vi "startup.vi"(8 "error in (no error)":errorcluster, 9 "deviceDataBase":refnum<class "deviceDataBase.lvclass">, 10 "HWControllerEvents":refnum<class "HWControllerEvents.lvclass">, 11 "Compiler in":refnum<class "Compiler.lvclass">) -> (0 "error out":errorcluster, 3 "Compiler out":refnum<class "Compiler.lvclass">)   [LabVIEW 2009, in "Compiler.lvlib" / "Compiler.lvclass"]
uses:
  Compiler.lvclass
  Hal/HWController/HWControllerEvents/HWControllerEvents.lvclass
  DatabaseHelpers/DbConnection/DeviceDataBase/deviceDataBase.lvclass
  Filing/FileSystem/FileSystem.lvclass
  Compiler.lvclass/Compiler.ctl
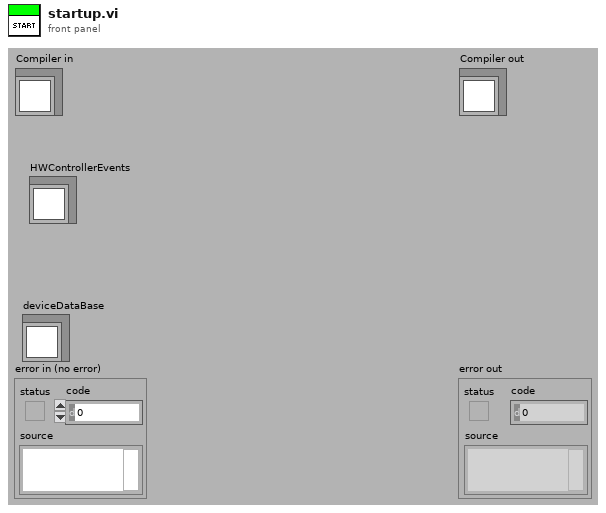
[diagram p1: front panel]
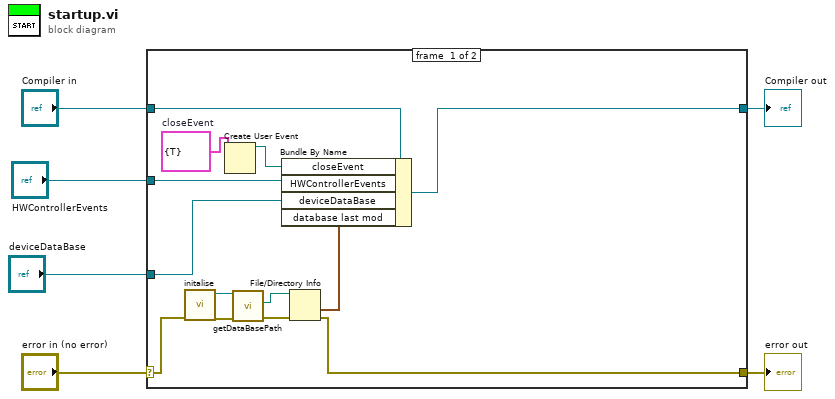
[diagram p0: block diagram]
diagram:
  n1 = case shown="No Error" "error in (no error)" {
    selector: "error in (no error)" -> [w10 w21]
    tunnel: [w9 w21] -> w5
    tunnel: [w16 w20] -> w3
    tunnel: "Compiler in" -> [w17 w20]
    tunnel: "HWControllerEvents" -> [w19 _]
    tunnel: "deviceDataBase" -> [w18 _]
    frame #0 {
      w8 = cluster{"close":bool} {"close"=TRUE}  # closeEvent
      n2 = call "initalise.vi"("error in (no error)"=w10) -> ("error out"=w14:errorcluster, "FileSystem out"=w15:refnum<class "FileSystem.lvclass">)  [unwired: 9 in]
      n3 = Create User Event(user event datatype=w8) -> (user event=w7:refnum<user-event>)  [unwired: 1 in, 1 out]
      n4 = call-dynamic "getDataBasePath.vi"("error in (no error)"=w14, "FileSystem.lvclass in"=w15) -> ("error out"=w12:errorcluster, "DataBasePath"=w13:path)  [unwired: 7 in, 1 out]
      n5 = File/Directory Info(path=w13, error in=w12) -> (last mod=w11:timestamp, error out=w9:errorcluster)  [unwired: 5 out]
      n6 = Bundle By Name(cluster=w17, "closeEvent"=w7, "HWControllerEvents"=w19, "deviceDataBase"=w18, "database last mod"=w11) -> (w16:refnum<class "Compiler.lvclass">)
    }
    frame #1 {
    }
  }
  "error out" <- w5
  "Compiler out" <- w3
